vi "Stop Core.vi"(10 "final error code":i32, 11 "Function in":refnum<class "Function.lvclass">) -> (3 "Function out":refnum<class "Function.lvclass">)   [LabVIEW 2016, in "Function Actor.lvlib" / "Function.lvclass"]
uses:
  <userlib>/Common Components/Function Actor/Function.lvclass
  <vilib>/event_ctls.llb/usereventprio.ctl
  <userlib>/Common Components/Function Actor/Function.lvclass/Function.ctl
  <vilib>/ActorFramework/Actor/Actor.lvclass
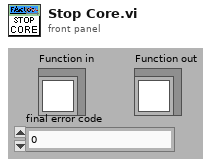
[diagram p1: front panel]
types:
  T1 = typedef "usereventprio.ctl" = enum32{"high priority", "normal priority"}
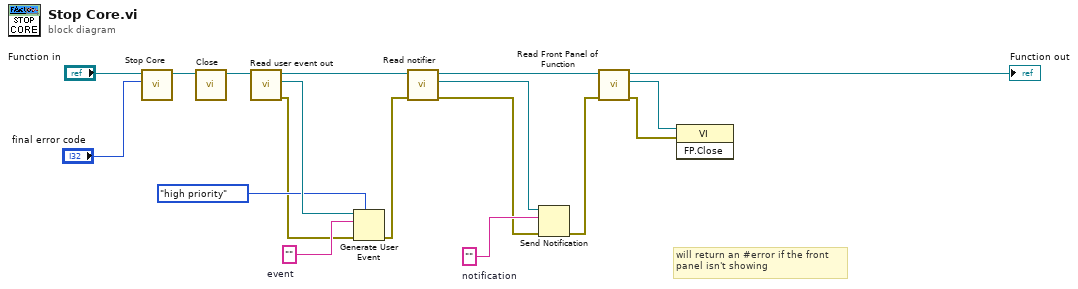
[diagram p0: block diagram]
diagram:
  w5 = ""  # event
  w16 = ""  # notification
  # "will return an #error if the front \npanel isn't showing"
  n1 = call-parent "Stop Core.vi"("final error code"="final error code", "Actor in"="Function in") -> ("Actor out"=w8:refnum<class "Function.lvclass">)  [unwired: 9 in]
  n2 = call-dynamic "Close.vi"("Function in"=w8) -> ("Function out"=w1:refnum<class "Function.lvclass">)  [unwired: 9 in, 1 out]
  n3 = call <userlib>:"Read user event out.vi"("Function in"=w1) -> ("error out"=w4:errorcluster, "user event out"=w7:refnum<user-event>, "Function out"=w9:refnum<class "Function.lvclass">)  [unwired: 8 in]
  n4 = Generate User Event(priority (normal)=usereventprio."high priority", user event=w7, event data cluster=w5, error in=w4) -> (error out=w3:errorcluster)  [unwired: 1 out]
  n5 = call <userlib>:"Read notifier.vi"("error in (no error)"=w3, "Function in"=w9) -> ("error out"=w12:errorcluster, "notifier"=w17:refnum<notifier>, "Function out"=w13:refnum<class "Function.lvclass">)  [unwired: 7 in]
  n6 = Send Notification(notification=w16, notifier=w17, error in (no error)=w12) -> (error out=w11:errorcluster)  [unwired: 1 out]
  n7 = call <userlib>:"Read Front Panel of Function.vi"("error in (no error)"=w11, "Function in"=w13) -> ("error out"=w2:errorcluster, "Front Panel of Function"=w10:refnum<vi>, "Function out"=→"Function out":refnum<class "Function.lvclass">)  [unwired: 7 in]
  n8 = invoke class="VI" method="FP.Close"(reference=w10, error in=w2) -> ()  [unwired: 1 in, 3 out]
